vi "DAQ_PW_Initial_before_Stream.vi"(8 "error in (no error)":errorcluster, 11 "USB_DEV_IN":string) -> (0 "error out":errorcluster, 1 "Vbat":dbl format="%0.5f", 2 "Vsource":dbl format="%0.5f", 3 "Refnum out":refnum<k21>)   [LabVIEW 2015]
uses:
  uPower-Kit2/Range_Shunt_selector.ctl
panel:
  in  "RANGE":string
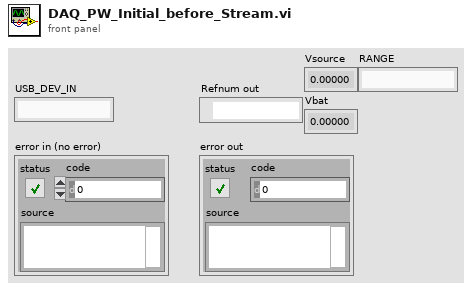
[diagram p1: front panel]
types:
  T1 = typedef "Range_Shunt_selector.ctl" = enum16{"uA Range  Rs = 3.3ohm", "mA Range Rs = 3.3ohm", "mA Range Rs = 1ohm", "mA Range Rs = 1ohm - X2"}
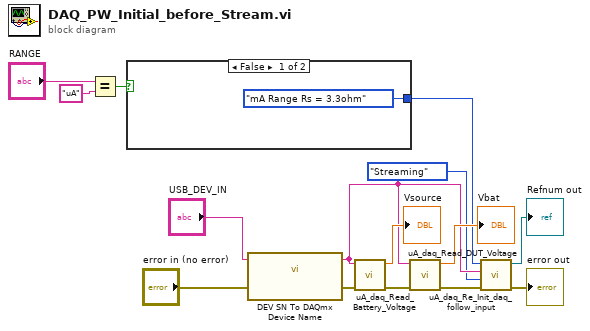
[diagram p0: block diagram]
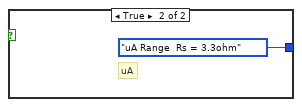
[diagram p2: hidden frame]
diagram:
  n1 = Equal?(x="RANGE", y="uA") -> (x = y?=w5:bool)
  n2 = case shown="False" w5 {
    tunnel: [Range_Shunt_selector."mA Range Rs = 3.3ohm" ("Range_shunt") Range_Shunt_selector."uA Range  Rs = 3.3ohm" ("Range_shunt")] -> w4
    frame False {
    }
    frame True {
      # "uA"
    }
  }
  n3 = call "DEV SN To DAQmx Device Name.vi"("error in (no error)"="error in (no error)", "USN_DEV (JSON)"="USB_DEV_IN") -> ("error out"=w12:errorcluster, "DAQmx Device Name"=w9:tag)  [unwired: 8 in]
  n4 = call "uA_daq_Read_Battery_Voltage.vi"("error in"=w12, "USB DAQ"=w9) -> ("error out"=w10:errorcluster, "Battery_Voltage"=→"Vsource":dbl)  [unwired: 8 in]
  n5 = call "uA_daq_Read_DUT_Voltage.vi"("error in"=w10, "USB DAQ"=w9) -> ("error out"=w3:errorcluster, "DUT_Voltage"=→"Vbat":dbl)  [unwired: 8 in]
  n6 = call "uA_daq_Re_Init_daq_follow_input.vi"("error in (no error)"=w3, "Acquire Mode"=enum16{"Streaming", "Read All", "Stop"}."Streaming", "USB"=w9, "Range_shunt"=w4) -> ("error out"=→"error out":errorcluster, "Refnum out"=→"Refnum out":refnum<k21>)  [unwired: 6 in]
